vi "H036 Harsh Pandit SCADA Lab 1a Sem 6.vi"() -> ()   [LabVIEW 2018]
panel:
  out "Temperature in F":dbl(slide) scale=0.0..100.0
  in  "Temperature in C":dbl(slide) scale=0.0..100.0
  # "Experiment 1a: Write a program to develope a program \nto convert the temperature from celsius to fahrenheit."
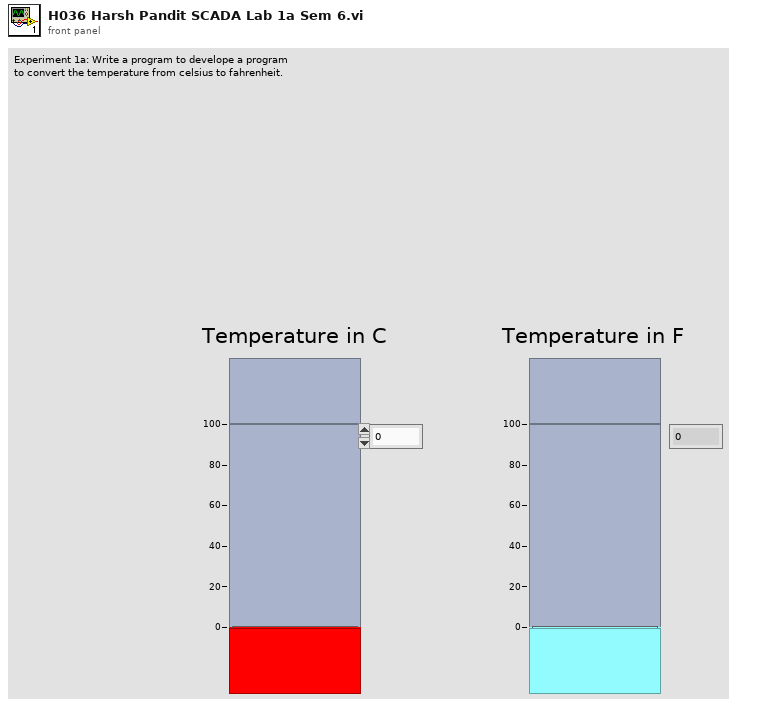
[diagram p1: front panel]
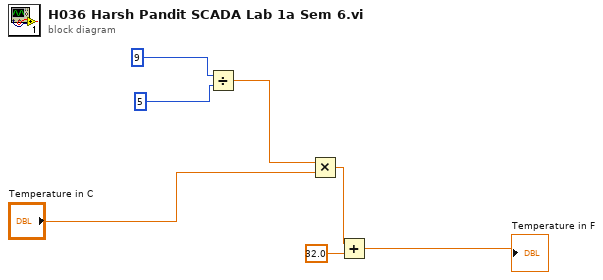
[diagram p0: block diagram]
diagram:
  n1 = Divide(x=9, y=5) -> (x/y=w5:dbl)
  n2 = Multiply(x=w5, y="Temperature in C") -> (x*y=w3:dbl)
  n3 = Add(x=w3, y=32.0) -> (x+y=→"Temperature in F":dbl)
